vi "Destroy.vi"(0 "reference in":refnum<class "Pgui_Obj.lvclass">, 5 "error in (no error)":errorcluster) -> (14 "reference out":refnum<class "Pgui_Obj.lvclass">, 19 "error out":errorcluster)   [LabVIEW 2019, in "Pgui_Obj.lvclass"]
uses:
  Pgui_Obj.lvclass
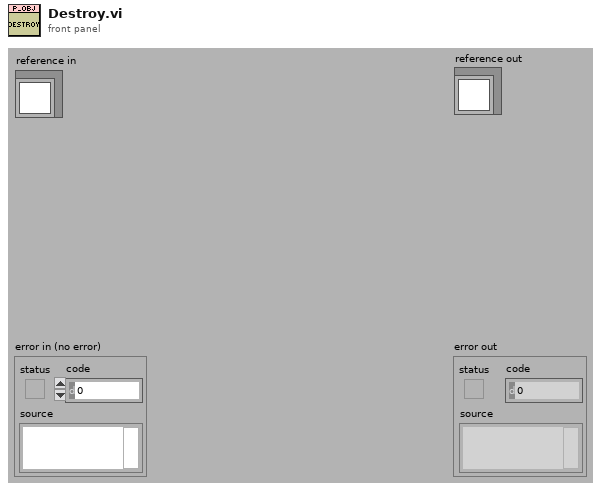
[diagram p1: front panel]
types:
  T1 = typedef "Pgui_Obj.lvclass/ObjectAttributes.ctl" = cluster{"Children":refnum<class "Pgui_Obj.lvclass">[], "Draw Instr":picture, "Params":cluster{"left":i16, "top":i16, "right":i16, "bottom":i16}, "Parent_Pgui_Obj":refnum<class "Pgui_Obj.lvclass">, "MouseOver":bool}
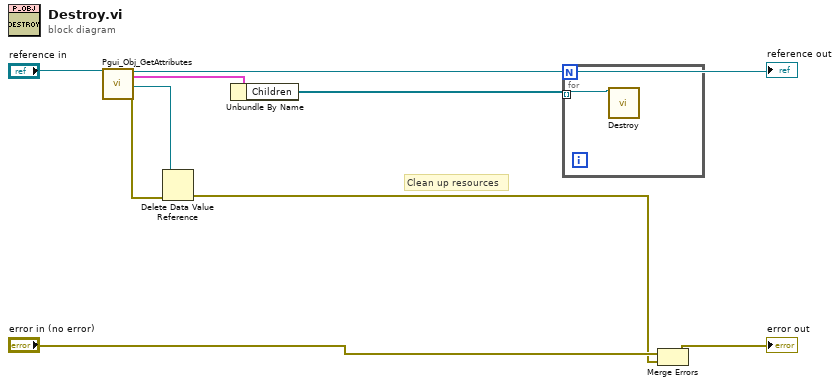
[diagram p0: block diagram]
diagram:
  # "Clean up resources"
  n1 = call "Pgui_Obj_GetAttributes.vi"("reference in"="reference in") -> ("reference out"=→"reference out":refnum<class "Pgui_Obj.lvclass">, "Data"=w2:T1, "DataRef"=w5:refnum<data-value>, "error out"=w6:errorcluster)  [unwired: 15 in]
  n2 = Delete Data Value Reference(data value reference=w5, error in=w6) -> (error out=w3:errorcluster)  [unwired: 1 out]
  n3 = Unbundle By Name(w2) -> ("Children"=w1:refnum<class "Pgui_Obj.lvclass">[])
  n4 = for {
    tunnel: w1 -> [w10] mode=indexing
    n5 = call-dynamic "Destroy.vi"("reference in"=w10) -> ()  [unwired: 17 in, 2 out]
  }
  n6 = Merge Errors("error in (no error)", w3) -> (→"error out":errorcluster)
